vi "GetWindowOpacity.vi"(8 "No Error":errorcluster, 11 "Window [SDL_Window *]":i64) -> (0 "error out":errorcluster, 3 "Opacity":sgl)   [LabVIEW 2024, in "SDL3.lvlib" / "Video.lvlib"]
doc: "<B>Summary</B>\nGet the opacity of a window.\n\n<B>Remarks</B>\nReturns the opacity, (0.0f - transparent, 1.0f - opaque).\nIf transparency isn't supported on this platform, opacity will be returned as 1.0f without error."
uses:
  Video.lvlib
  Error/Error.lvlib
  Lib/SDL3-32.dll
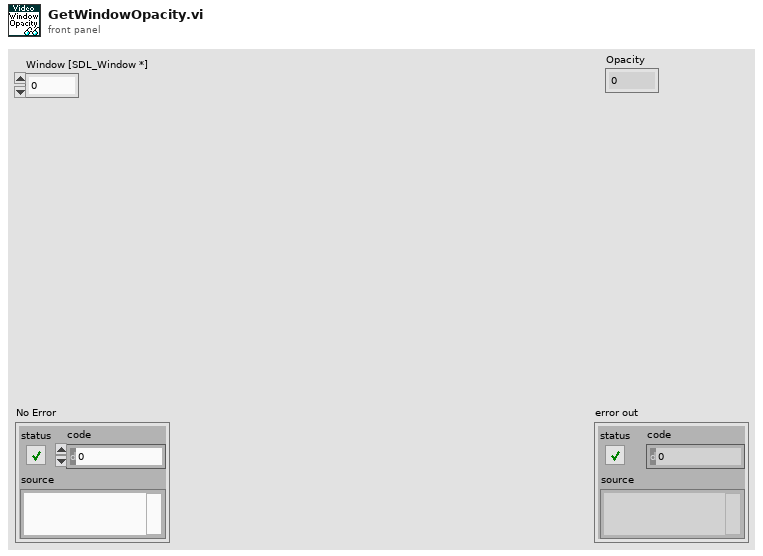
[diagram p1: front panel]
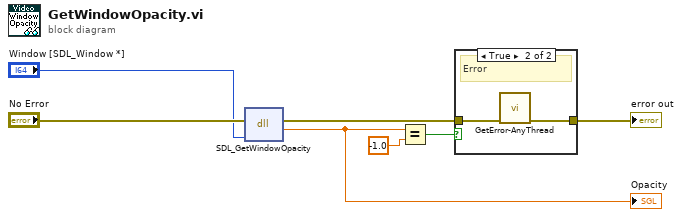
[diagram p0: block diagram]
diagram:
  n1 = dll-call lib="C:/Users/Thomas/Documents/Projects/LV-SDL3/Lib/SDL3-*.*" fn="SDL_GetWindowOpacity"(error in="No Error", "window"="Window [SDL_Window *]") -> (error out=w3:errorcluster, "return type"=w4:sgl)  [unwired: 3 in, 1 out]
  "Opacity" <- w4
  n2 = Equal?(x=w4, y=sgl -1.0) -> (x = y?=w2:bool)
  n3 = case shown="True" w2 {
    tunnel: w3 -> [w8 w10]
    tunnel: [w8 w9] -> w6
    frame False {
      # "Ok"
    }
    frame True {
      # "Error"
      n4 = call "GetError-AnyThread.vi"("No Error"=w10) -> ("Error Out"=w9:errorcluster)  [unwired: 10 in]
    }
  }
  "error out" <- w6
